vi "LibXML_TransformWithXSLT.vi"(8 "error in (no error)":errorcluster, 9 "Output-file":string, 10 "XML file":string, 11 "XSLT file":string) -> (0 "error out":errorcluster, 3 "bytes written":i32)   [LabVIEW 2019, in "Tools.lvlib" / "LibXML.lvlib"]
doc: "Transform XML from a file with XSLT and write to a new file."
uses:
  LibXML.lvlib
  dll/lXMLwrap.dll
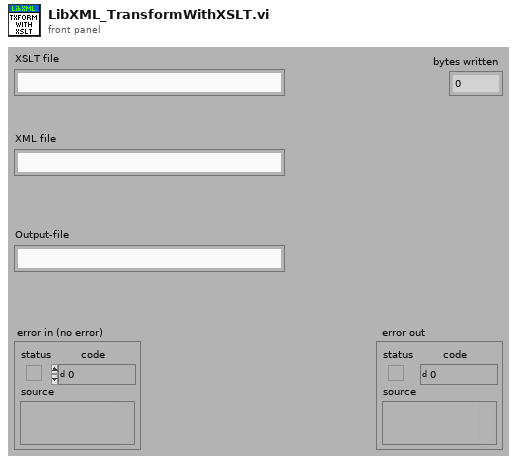
[diagram p1: front panel]
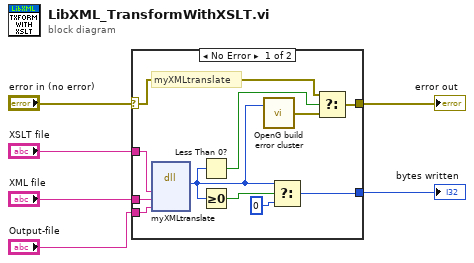
[diagram p0: block diagram]
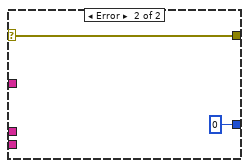
[diagram p2: hidden frame]
diagram:
  n1 = case shown="No Error" "error in (no error)" {
    selector: "error in (no error)" -> [w7 w19]
    tunnel: [w15 w19] -> w6
    tunnel: [w11 0 ("f")] -> w4
    tunnel: "XSLT file" -> [w10 _]
    tunnel: "XML file" -> [w9 _]
    tunnel: "Output-file" -> [w8 _]
    frame No Error {
      # "myXMLtranslate"
      n2 = dll-call lib="C:/Projects/_Prywatne/MyCIT/Framework/Tools/XML/LibXML/dll/lXMLwrap.dll" fn="myXMLtranslate"("XSLfile"=w10, "XMLfile"=w9, "outFile"=w8) -> ("return type"=w13:i32)  [unwired: 6 in, 2 out]
      n3 = Less Than 0?(x=w13) -> (x < 0?=w16:bool)
      n4 = Greater Or Equal To 0?(x=w13) -> (x >= 0?=w14:bool)
      n5 = call "OpenG build error cluster.vi"("code"=w13) -> ("error out"=w17:errorcluster)  [unwired: 1 in]
      n6 = Select(t=w13, s=w14, f=0) -> (s? t:f=w11:i32)
      n7 = Select(t=w7, s=w16, f=w17) -> (s? t:f=w15:errorcluster)
    }
    frame Error {
    }
  }
  "error out" <- w6
  "bytes written" <- w4
